vi "Close.vi"(8 "error in":errorcluster, 11 "Control Load CFG in":refnum<class "EL Control Load CFG.lvclass">) -> (0 "error out":errorcluster, 3 "Control Load CFG out":refnum<class "EL Control Load CFG.lvclass">)   [LabVIEW 2023, in "EL Control Load CFG.lvclass"]
uses:
  EL Control Load CFG.lvclass
  Configuration/Configuration Semaphore/CFG Semaphore.lvclass
  EL Control Load CFG.lvclass/EL Control Load CFG.ctl
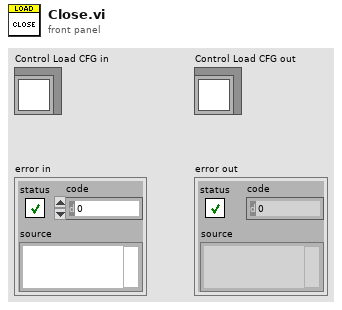
[diagram p1: front panel]
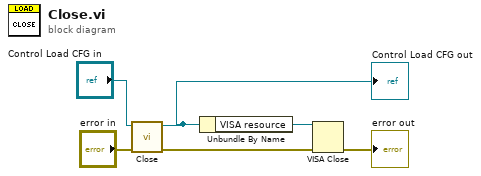
[diagram p0: block diagram]
diagram:
  n1 = call-parent "Close.vi"("error in"="error in", "CFG Semaphore in"="Control Load CFG in") -> ("error out"=w6:errorcluster, "CFG Semaphore out"=w3:refnum<class "EL Control Load CFG.lvclass">)  [unwired: 8 in]
  "Control Load CFG out" <- w3
  n2 = Unbundle By Name(w3) -> ("VISA resource"=w1:refnum<visa-resource-name>)
  n3 = VISA Close(VISA resource name=w1, error in (no error)=w6) -> (error out=→"error out":errorcluster)
